vi "Method.vi"(4 "Input B":refnum<class "Abs_Numeric.lvclass">, 5 "Input A":T1) -> (1 "Result":T1)   [LabVIEW 2021, in "Subtract_U8.lvclass"]
uses:
  Subtract_U8.lvclass
  Abs Type.ctl
  Abs_Types/U8 Integer/Abs_U8 Integer.lvclass
  Abs_Types/Numeric/Abs_Numeric.lvclass
  C:/Users/Tim/Documents/LabVIEW/2021/Data Classes/Source/Functions/Support/Two Terminal/U8/AbsFunc_Two Term_U8.lvclass
  C:/Users/Tim/Documents/LabVIEW/2021/Data Classes/Source/Abs_Types/U8 Integer/Abs_U8 Integer.lvclass
  Support/Two Terminal/U8/AbsFunc_Two Term_U8.lvclass/AbsFunc_Two Term_U8.ctl
  Support/Two Terminal/U8/Properties/Write Numeric A.vi
  Support/Two Terminal/U8/Properties/Write Numeric B.vi
  Subtract_U8.lvclass/Subtract_U8.ctl
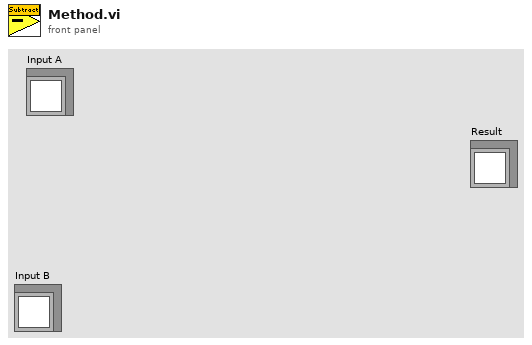
[diagram p1: front panel]
types:
  T1 = typedef "Subtract_U8.lvclass/Abs Type.ctl" = refnum<class "Abs_U8 Integer.lvclass">
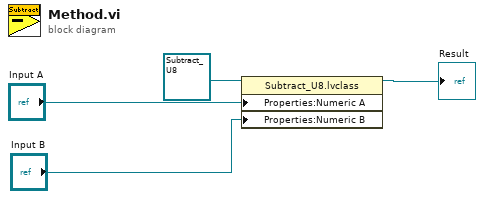
[diagram p0: block diagram]
diagram:
  n1 = property class="Subtract_U8.lvclass"(reference=refnum<class "Subtract_U8.lvclass"> refnum ("Subtract_DBL.lvclass"), "Properties:Numeric A"="Input A", "Properties:Numeric B"="Input B") -> (reference out=→"Result":refnum<class "Subtract_U8.lvclass">)  [unwired: 1 in, 1 out]
